vi "plotBoardCanvas.vi"(8 "error in (no error)":errorcluster, 11 "object in":refnum<class "Board.lvclass">) -> (0 "error out":errorcluster, 3 "object out":refnum<class "Board.lvclass">)   [LabVIEW 2020, in "Board.lvclass"]
doc: "Plots the board with the color pattern"
uses:
  Board.lvclass
  Board.lvclass/Board.ctl
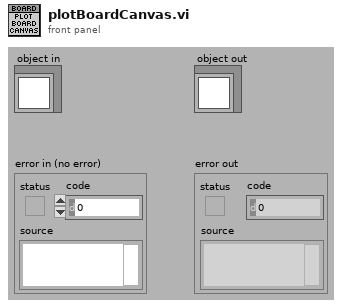
[diagram p1: front panel]
types:
  T1 = cluster{"left":i16, "top":i16, "right":i16, "bottom":i16}
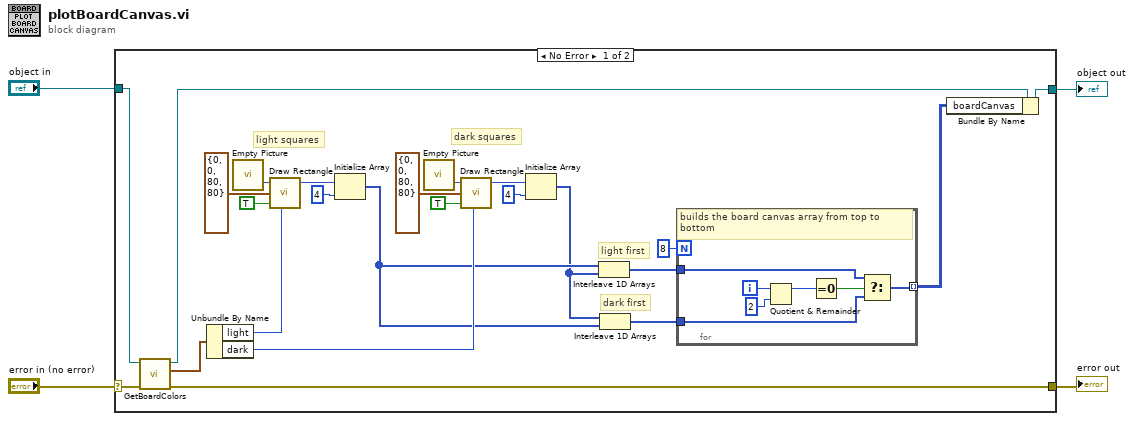
[diagram p0: block diagram]
diagram:
  n1 = case shown="No Error" "error in (no error)" {
    selector: "error in (no error)" -> [w28 w37]
    tunnel: [w27 w37] -> w3
    tunnel: [w6 w36] -> w1
    tunnel: "object in" -> [w26 w36]
    frame No Error {
      # "light first"
      # "dark first"
      # "dark squares"
      # "light squares"
      n2 = call "GetBoardColors.vi"("error in (no error)"=w28, "object in"=w26) -> ("error out"=w27:errorcluster, "boardColors"=w21:cluster{"light":u32, "dark":u32}, "object out"=w25:refnum<class "Board.lvclass">)  [unwired: 7 in]
      n3 = Unbundle By Name(w21) -> ("light"=w20:u32, "dark"=w16:u32)
      n4 = call "Empty Picture"() -> ("empty picture"=w24:picture)
      n5 = call <vilib>:"Draw Rectangle.vi"("picture"=w24, "rect"=T1 {"left"=0, "top"=0, "right"=80, "bottom"=80}, "fill?(F)"=TRUE, "color(black)"=w20) -> ("new picture"=w15:picture)  [unwired: 5 in]
      n6 = Initialize Array(w15, 4 ("dimension size")) -> (w10:picture[])
      n7 = call "Empty Picture"() -> ("empty picture"=w17:picture)
      n8 = call <vilib>:"Draw Rectangle.vi"("picture"=w17, "rect"=T1 {"left"=0, "top"=0, "right"=80, "bottom"=80}, "fill?(F)"=TRUE, "color(black)"=w16) -> ("new picture"=w12:picture)  [unwired: 5 in]
      n9 = Initialize Array(w12, 4 ("dimension size")) -> (w9:picture[])
      n10 = Interleave 1D Arrays(w10, w9) -> (w7:picture[])
      n11 = Interleave 1D Arrays(w9, w10) -> (w8:picture[])
      n12 = for {
        N: 8 -> [_]
        tunnel: w8 -> [w30]
        tunnel: w7 -> [w31]
        tunnel: [w29] -> w5 mode=indexing
        i -> [w35]
        # "builds the board canvas array from top to bottom"
        n13 = Quotient & Remainder(x=w35, y=2) -> (x-y*floor(x/y)=w34:i32)  [unwired: 1 out]
        n14 = Equal To 0?(x=w34) -> (x = 0?=w33:bool)
        n15 = Select(t=w31, s=w33, f=w30) -> (s? t:f=w29:picture[])
      }
      n16 = Bundle By Name(cluster=w25, "boardCanvas"=w5) -> (w6:refnum<class "Board.lvclass">)
    }
    frame Error {
    }
  }
  "error out" <- w3
  "object out" <- w1
